vi "Turbomolecular Pressure.vi"(6 "Tube Radius (mm)":dbl=1.2192, 8 "Temperature Cold (K)":dbl, 9 "Temperature Warm (K)":dbl, 10 "Pressure Cold (mbar)":dbl, 11 "Pressure Warm (mbar)":dbl) -> (3 "Pressure Function":dbl)   [LabVIEW 2019]
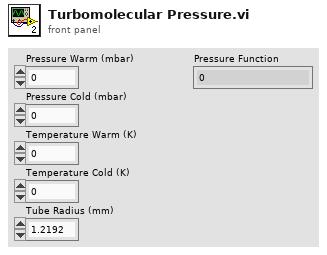
[diagram p1: front panel]
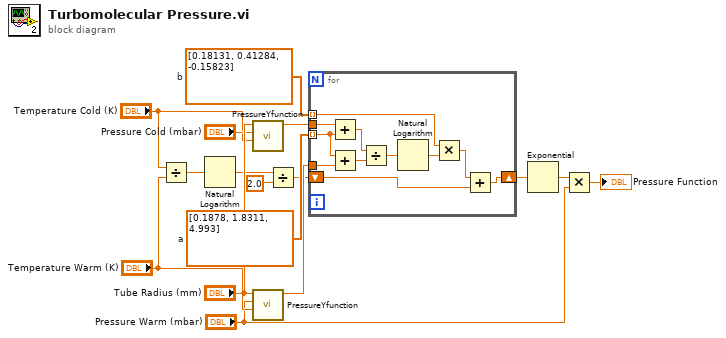
[diagram p0: block diagram]
diagram:
  w6 = dbl[] [0.18131, 0.41284, -0.15823]  # b
  w9 = dbl[] [0.1878, 1.8311, 4.993]  # a
  n1 = Divide(x="Temperature Cold (K)", y="Temperature Warm (K)") -> (x/y=w12:dbl)
  n2 = Natural Logarithm(1:w12) -> (0:w11:dbl)
  n3 = call "PressureYfunction.vi"("Temperature (K)"="Temperature Cold (K)", "Pressure (mbar)"="Pressure Cold (mbar)", "Tube Radius (mm)"="Tube Radius (mm)") -> ("Y(r,p,t)"=w7:dbl)  [unwired: 8 in]
  n4 = call "PressureYfunction.vi"("Temperature (K)"="Temperature Warm (K)", "Pressure (mbar)"="Pressure Warm (mbar)", "Tube Radius (mm)"="Tube Radius (mm)") -> ("Y(r,p,t)"=w8:dbl)  [unwired: 8 in]
  n5 = Divide(x=w11, y=2.0) -> (x/y=w5:dbl)
  n6 = for {
    tunnel: w9 -> [w25] mode=indexing
    tunnel: w8 -> [w27]
    tunnel: w7 -> [w26]
    tunnel: w6 -> [w20] mode=indexing
    shift-right: [w17] -> w4
    shift-left: w5 -> [w18]
    n7 = Add(x=w26, y=w25) -> (x+y=w24:dbl)
    n8 = Add(x=w25, y=w27) -> (x+y=w23:dbl)
    n9 = Divide(x=w24, y=w23) -> (x/y=w22:dbl)
    n10 = Natural Logarithm(1:w22) -> (0:w21:dbl)
    n11 = Multiply(x=w20, y=w21) -> (x*y=w19:dbl)
    n12 = Add(x=w19, y=w18) -> (x+y=w17:dbl)
  }
  n13 = Exponential(1:w4) -> (0:w3:dbl)
  n14 = Multiply(x=w3, y="Pressure Warm (mbar)") -> (x*y=→"Pressure Function":dbl)
